vi "BaggingRegressor.vi"(8 "error in":errorcluster) -> (0 "error out":errorcluster, 3 "out":refnum<class "BaggingRegressor.lvclass">)   [LabVIEW 2020]
doc: "A Bagging regressor.\n\n A Bagging regressor is an ensemble meta-estimator that fits base\n regressors each on random subsets of the original dataset and then\n aggregate their individual predictions (either by voting or by averaging)\n to form a final prediction. Such a meta-estimator can typically be used as\n a way to reduce the variance of a black-box estimator (e.g., a decision\n tree), by introducing randomization into its construction procedure and\n then making an ensemble out of it.\n\n This algorithm encompasses several works from the literature. When random\n subsets of the dataset are drawn as random subsets of the samples, then\n this algorithm is known as Pasting [1]_. If samples are drawn with\n replacement, then the method is known as Bagging [2]_. When random subsets\n of the dataset are drawn as random subsets of the features, then the method\n is known as Random Subspaces [3]_. Finally, when base estimators are built\n on subsets of both samples and features, then the method is known as\n Random Patches [4]_.\n\n Read more in the :ref:`User Guide <bagging>`.\n\n .. versionadded:: 0.15\n\n Parameters\n ----------\n base_estimator : object, default=None\n The base estimator to fit on random subsets of the dataset.\n If None, then the base estimator is a\n :class:`~sklearn.tree.DecisionTreeRegressor`.\n\n n_estimators : int, default=10\n The number of base estimators in the ensemble.\n\n max_samples : int or float, default=1.0\n The number of samples to draw from X to train each base estimator (with\n replacement by default, see `bootstrap` for more details).\n\n - If int, then draw `max_samples` samples.\n - If float, then draw `max_samples * X.shape[0]` samples.\n\n max_features : int or float, default=1.0\n The number of features to draw from X to train each base estimator (\n without replacement by default, see `bootstrap_features` for more\n details).\n\n - If int, then draw `max_features` features.\n - If float, then draw `max_features * X.shape[1]` features.\n\n bootstrap : bool, default=True\n Whether samples are drawn with replacement. If False, sampling\n without replacement is performed.\n\n bootstrap_features : bool, default=False\n Whether features are drawn with replacement.\n\n oob_score : bool, default=False\n Whether to use out-of-bag samples to estimate\n the generalization error. Only available if bootstrap=True.\n\n warm_start : bool, default=False\n When set to True, reuse the solution of the previous call to fit\n and add more estimators to the ensemble, otherwise, just fit\n a whole new ensemble. See :term:`the Glossary <warm_start>`.\n\n n_jobs : int, default=None\n The number of jobs to run in parallel for both :meth:`fit` and\n :meth:`predict`. ``None`` means 1 unless in a\n :obj:`joblib.parallel_backend` context. ``-1`` means using all\n processors. See :term:`Glossary <n_jobs>` for more details.\n\n random_state : int, RandomState instance or None, default=None\n Controls the random resampling of the original dataset\n (sample wise and feature wise).\n If the base estimator accepts a `random_state` attribute, a different\n seed is generated for each instance in the ensemble.\n Pass an int for reproducible output across multiple function calls.\n See :term:`Glossary <random_state>`.\n\n verbose : int, default=0\n Controls the verbosity when fitting and predicting.\n\n Attributes\n ----------\n base_estimator_ : estimator\n The base estimator from which the ensemble is grown.\n\n n_features_ : int\n The number of features when :meth:`fit` is performed.\n\n estimators_ : list of estimators\n The collection of fitted sub-estimators.\n\n estimators_samples_ : list of arrays\n The subset of drawn samples (i.e., the in-bag samples) for each base\n estimator. Each subset is defined by an array of the indices selected.\n\n estimators_features_ : list of arrays\n The subset of drawn features for each base estimator.\n\n oob_score_ : float\n Score of the training dataset obtained using an out-of-bag estimate.\n This attribute exists only when ``oob_score`` is True.\n\n oob_prediction_ : ndarray of shape (n_samples,)\n Prediction computed with out-of-bag estimate on the training\n set. If n_estimators is small it might be possible that a data point\n was never left out during the bootstrap. In this case,\n `oob_prediction_` might contain NaN. This attribute exists only\n when ``oob_score`` is True.\n\n \nAvailable methods:\nFit\nPredict\nScore\nGet Attributes\nGet Params\nSet Params"
uses:
  BaggingRegressor.lvclass
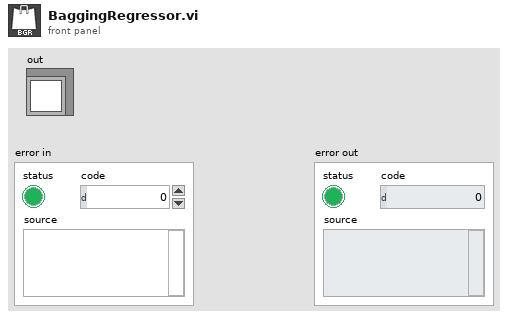
[diagram p1: front panel]
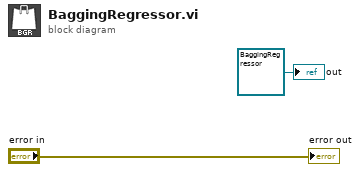
[diagram p0: block diagram]
diagram:
  "out" <- refnum<class "BaggingRegressor.lvclass"> refnum ("model")
  "error out" <- "error in"
